vi "for.vi"() -> ()   [LabVIEW 2020]
panel:
  out "Thermometer":dbl(slide) scale=0.0..100.0
  out "Numeric":i32
  # "for"
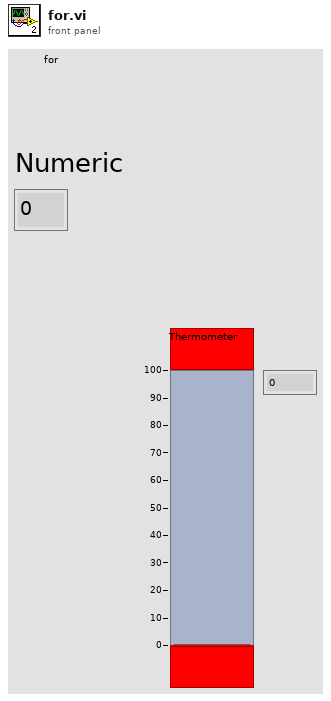
[diagram p1: front panel]
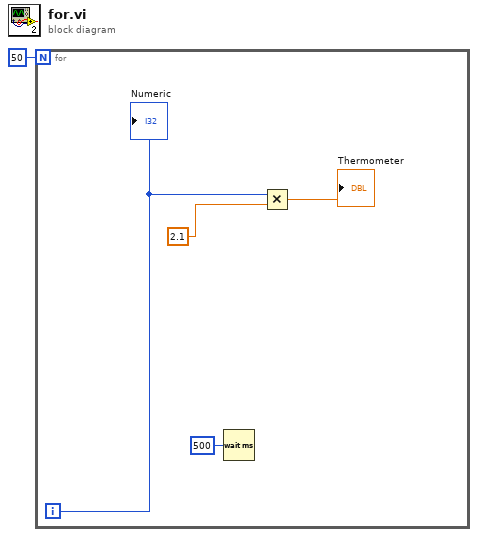
[diagram p0: block diagram]
diagram:
  n1 = for {
    N: 50 -> [_]
    i -> [w4]
    n2 = Wait (ms)(milliseconds to wait=u32 500) -> ()  [unwired: 1 out]
    n3 = Multiply(x=w4, y=2.1) -> (x*y=→"Thermometer":dbl)
    "Numeric" <- w4
  }
